vi "Disconnect.vi"(8 "error in":errorcluster, 11 "LTB-1 in":refnum<class "LTB-1.lvclass">) -> (0 "error out":errorcluster, 3 "LTB-1 out":refnum<class "LTB-1.lvclass">)   [LabVIEW 2018, in "LTB-1.lvlib" / "LTB-1.lvclass"]
doc: "This is the parent class, the child class will override the function and use the appropriate methods to disconnect from the unit.\n\nAuthor: Ron Dexter\nCompany: Luminar\nModified: 5/20/2018"
uses:
  LTB-1.lvclass
  C:/AME Test Engineering/LabVIEW/PPLs/EXFO/Parent/EXFO.lvlibp/EXFO.lvclass
  PPLs/EXFO/Parent/EXFO.lvlibp/Methods/Read Resource.vi
  3150 Driver/3150.lvlib
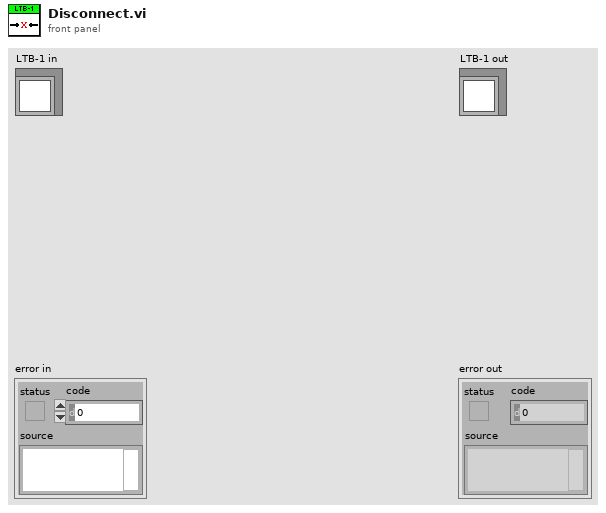
[diagram p1: front panel]
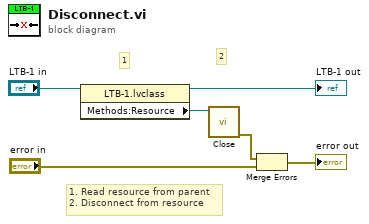
[diagram p0: block diagram]
diagram:
  # "2"
  # "1"
  # "1. Read resource from parent\n2. Disconnect from resource"
  n1 = property class="LTB-1.lvclass"(reference="LTB-1 in") -> (reference out=→"LTB-1 out":refnum<class "LTB-1.lvclass">, "Methods:Resource"=w2:refnum<visa-resource-name>)  [unwired: 1 in, 1 out]
  n2 = call "Close.vi"("VISA resource name"=w2) -> ("error out"=w1:errorcluster)  [unwired: 10 in]
  n3 = Merge Errors(w1, "error in") -> (→"error out":errorcluster)
